vi "Shared Variables Tester.vi"() -> ()   [LabVIEW 2013]
doc: "Tester for the Shared Variables API"
uses:
  FA_SharedVariables.ctl
  FA_NativeTypes API/source/VI Source/FA_Config.ctl
  FA_LocalStore API/source/VI Source/FA_LSSpecialTypes.ctl
  FA_SharedVariables.lvlib
  FA_NativeTypes API/source/VI Source/FA_NativeTypes.lvlib
  FA_LocalStore API/source/VI Source/FA_LocalStore.lvlib
panel:
  out "Config":T1
  in  "error in (no error)":errorcluster
  out "error out":errorcluster
  out "SV":T3
  in  "XML String":string="<?xml version=\"1.0\" encoding=\"UTF-8\"?>\n<Config>\r\n  <Id>myID</Id>\r\n  <Name>Shared Variables</Name>\r\n  <Parameter>\r\n    <Name>0.Type</Name>\r\n    <Value>myType</Value>\r\n  </Parameter>\r\n  <Parameter>\r\n    <Name>1.URL</Name>\r\n    <Value>myURL</Value>\r\n  </Parameter>\r\n  <Parameter>\r\n    <Name>2.Type</Name>\r\n    <Value>myType2</Value>\r\n  </Parameter>\r\n  <Parameter>\r\n    <Name>3.URL</Name>\r\n    <Value>myURL2</Value>\r\n  </Parameter>\r\n  <Account>myAccount</Account>\r\n  <CreateDate>now</CreateDate>\r\n  <LastModified>then</LastModified>\r\n</Config>"
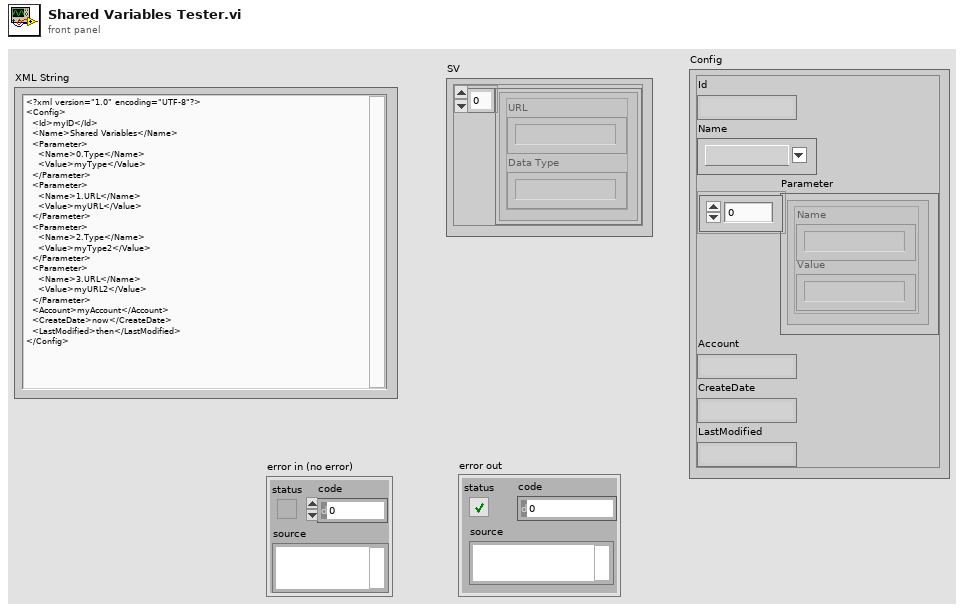
[diagram p1: front panel]
types:
  T1 = typedef "FA_NativeTypes.lvlib/FA_Config.ctl" = cluster{"Id":string, "Name":T2, "Parameter":cluster{"Name":string, "Value":string}[], "Account":string, "CreateDate":string, "LastModified":string}
  T2 = typedef "FA_LocalStore.lvlib/FA_LSSpecialTypes.ctl" = string
  T3 = typedef "FA_SharedVariables.lvlib/FA_SharedVariables.ctl" = cluster{"Shared Variables":cluster{"URL":string, "Data Type":string}[]}
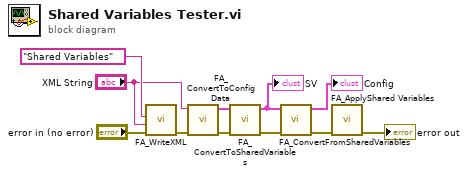
[diagram p0: block diagram]
diagram:
  n1 = call "FA_WriteXML.vi"("Error In"="error in (no error)", "XML String"="XML String", "Special Type"=T2 "Shared Variables") -> ("Error Out"=w3:errorcluster)  [unwired: 6 in]
  n2 = call "FA_ConvertToConfigData.vi"("Error In"=w3, "XML String"="XML String") -> ("Error Out"=w9:errorcluster, "ConfigData"=w8:T1)  [unwired: 8 in]
  n3 = call "FA_ConvertToSharedVariables.vi"("Error In"=w9, "Config"=w8) -> ("Error Out"=w11:errorcluster, "SV"=w10:T3)  [unwired: 8 in]
  "SV" <- w10
  n4 = call "FA_ConvertFromSharedVariables.vi"("Error In"=w11, "Shared Variable"=w10) -> ("Error Out"=w7:errorcluster, "Config"=→"Config":T1)  [unwired: 8 in]
  n5 = call "FA_ApplyShared Variables.vi"("Error In"=w7) -> ("Error Out"=→"error out":errorcluster)  [unwired: 10 in]
